vi "Empty Tree.vi"(8 "error in (no error)":errorcluster, 11 "Tree ref in":refnum<vi>) -> (0 "error out":errorcluster)   [LabVIEW 2021, in "CIF_UI.lvclass"]
uses:
  CIF_UI.lvclass
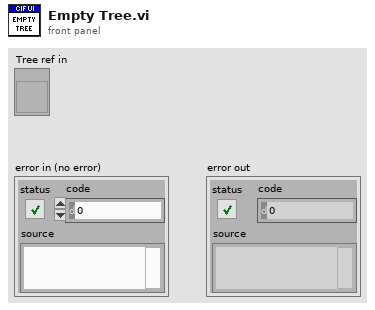
[diagram p1: front panel]
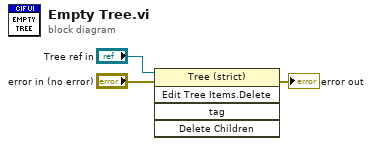
[diagram p0: block diagram]
diagram:
  n1 = invoke class="Tree (strict)" method="Edit Tree Items.Delete"(reference="Tree ref in", error in="error in (no error)") -> (error out=→"error out":errorcluster)  [unwired: 3 in, 4 out]
